vi "TestRUSHShoot.vi"() -> ()   [LabVIEW 2012]
panel:
  in  "ShootConstElev":cluster{"1":dbl, "2":dbl, "3":dbl}={"1"=45.0, "2"=24.0, "3"=12.0}
  in  "ShootTargetInfo":T1
  in  "Deadband":dbl=0.1
  in  "Default Wheel Speed":dbl=0.75
  in  "IndexerSpeed":dbl=0.5
  in  "ShootManualElev":dbl(slide) scale=-1.0..1.0
  in  "ShootPOTElev":dbl(slide) scale=0.0..45.0
  in  "ShootSetElev":dbl
  in  "ShootIndexerEnable":bool
  in  "ShootStartWheels":bool
  in  "ShootTrackEnable":bool
  out "Out Cluster":T2
  in  "In Cluster":T3
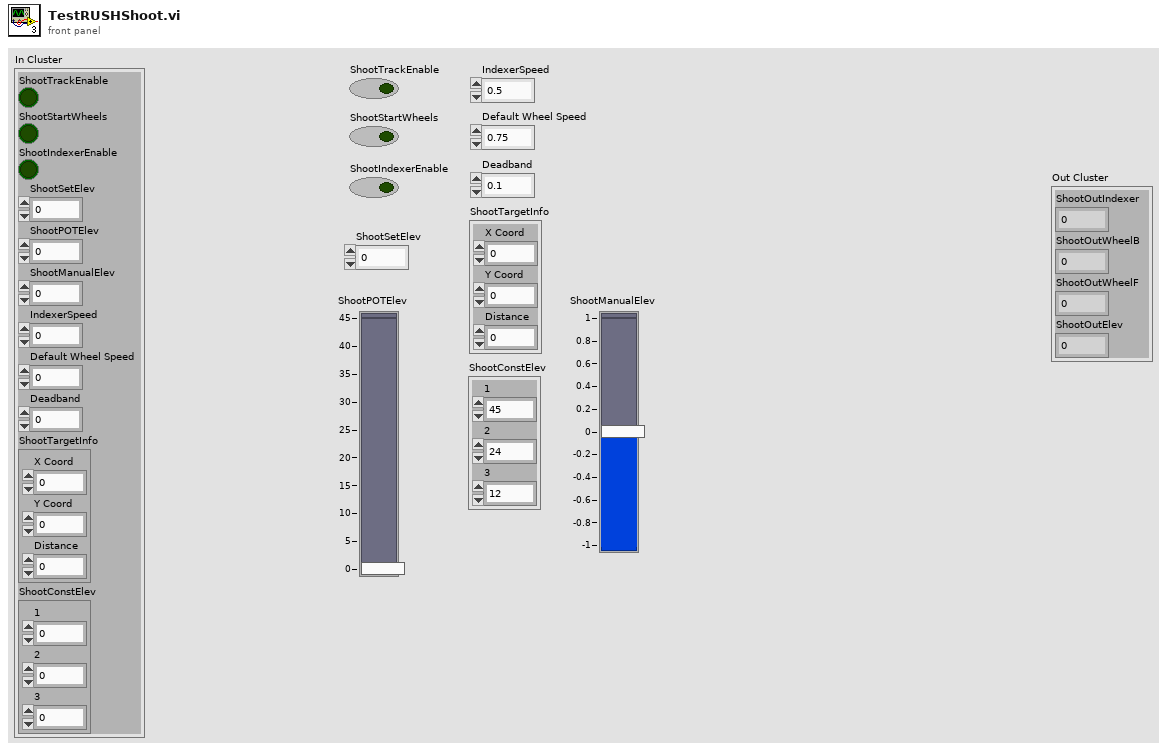
[diagram p1: front panel]
types:
  T1 = cluster{"X Coord":dbl, "Y Coord":dbl, "Distance":dbl}
  T2 = cluster{"ShootOutIndexer":dbl, "ShootOutWheelB":dbl, "ShootOutWheelF":dbl, "ShootOutElev":dbl}
  T3 = cluster{"ShootTrackEnable":bool, "ShootStartWheels":bool, "ShootIndexerEnable":bool, "ShootSetElev":dbl, "ShootPOTElev":dbl, "ShootManualElev":dbl, "IndexerSpeed":dbl, "Default Wheel Speed":dbl, "Deadband":dbl, "ShootTargetInfo":cluster{"X Coord":dbl, "Y Coord":dbl, "Distance":dbl}, "ShootConstElev":cluster{"1":dbl, "2":dbl, "3":dbl}}
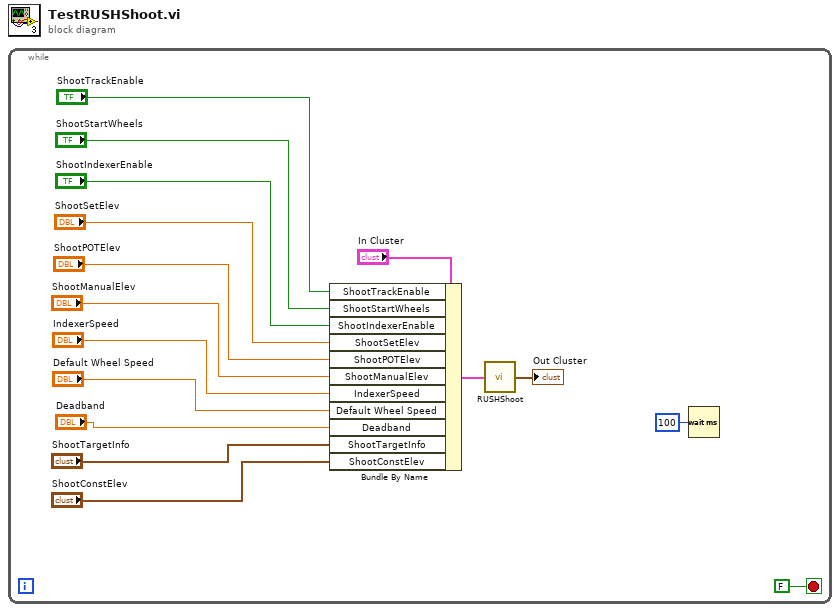
[diagram p0: block diagram]
diagram:
  n1 = while {
    stop <- FALSE stop-if-true
    n2 = Bundle By Name(cluster="In Cluster", "ShootTrackEnable"="ShootTrackEnable", "ShootStartWheels"="ShootStartWheels", "ShootIndexerEnable"="ShootIndexerEnable", "ShootSetElev"="ShootSetElev", "ShootPOTElev"="ShootPOTElev", "ShootManualElev"="ShootManualElev", "IndexerSpeed"="IndexerSpeed", "Default Wheel Speed"="Default Wheel Speed", "Deadband"="Deadband", "ShootTargetInfo"="ShootTargetInfo", "ShootConstElev"="ShootConstElev") -> (w15:T3)
    n3 = call "RUSHShoot.vi"("In Cluster"=w15) -> ("Out Cluster"=→"Out Cluster":T2)
    n4 = Wait (ms)(milliseconds to wait=u32 100) -> ()  [unwired: 1 out]
  }
